vi "Mandar datos.vi"() -> ()   [LabVIEW 2020]
uses:
  <vilib>/httpClient/PUTBuffer.vi
  <vilib>/httpClient/LabVIEWHTTPClient.lvlib
panel:
  out "error out":errorcluster
  out "headers Put":string
  out "body PUT":string
  in  "stop":bool
  in  "Dial":dbl(knob) scale=0.0..10.0
  in  "Led rele":bool
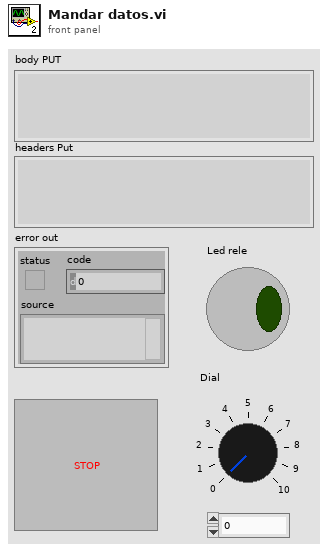
[diagram p1: front panel]
types:
  T1 = cluster{"Acondicionamiento":dbl, "Data":string, "Hora":string, "Led rele":bool}
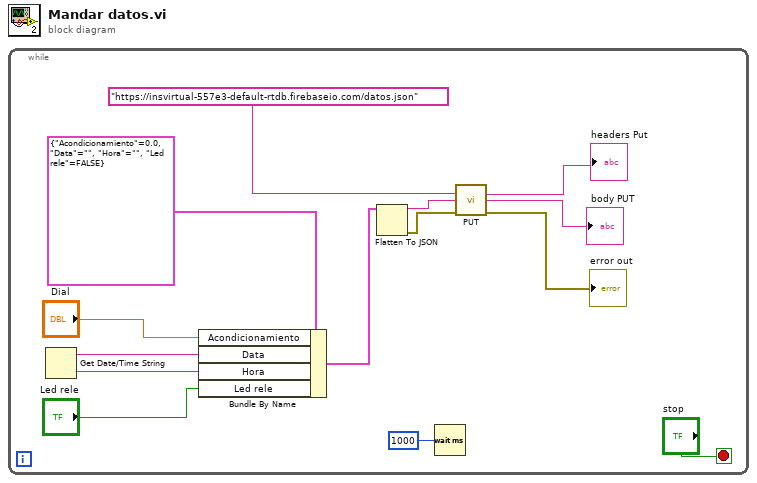
[diagram p0: block diagram]
diagram:
  n1 = while {
    stop <- "stop" stop-if-true
    n2 = Get Date/Time String() -> (date string=w10:string, time string=w6:string)  [unwired: 3 in]
    n3 = Bundle By Name(cluster=T1 {"Acondicionamiento"=0.0, "Data"="", "Hora"="", "Led rele"=FALSE}, "Acondicionamiento"="Dial", "Data"=w10, "Hora"=w6, "Led rele"="Led rele") -> (w7:T1)
    n4 = Flatten To JSON(anything=w7) -> (JSON string=w3:string, 11:w2:errorcluster)  [unwired: 2 in]
    n5 = Wait (ms)(milliseconds to wait=u32 1000) -> ()  [unwired: 1 out]
    n6 = call-poly <vilib>:"PUT.vi"("url"="https://insvirtual-557e3-default-rtdb.firebaseio.com/datos.json", "buffer"=w3, "error in (no error)"=w2) -> ("headers"=→"headers Put":string, "body"=→"body PUT":string, "error out"=→"error out":errorcluster)  [unwired: 9 in, 1 out]
  }
